vi "manage_objectives.vi"(8 "error in (no error)":errorcluster) -> (0 "error out":errorcluster)   [LabVIEW 2010]
uses:
  components/Objective/GenericObjective/GenericObjective/GenericObjective.lvclass
panel:
  in  "renameButton":bool
  in  "deleteButton":bool
  in  "editButton":bool
  in  "doneButton":bool
  in  "createButton":bool
  in  "new configuration":string
  in  "existing configurations":i32(listbox)
  # "Manage objectives"
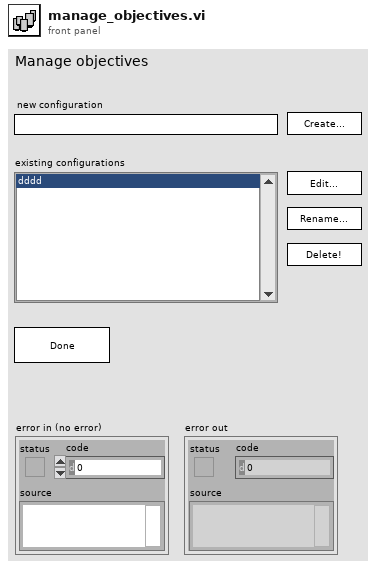
[diagram p1: front panel]
types:
  T1 = enum8{"Enabled", "Disabled", "Disabled and Grayed Out"}
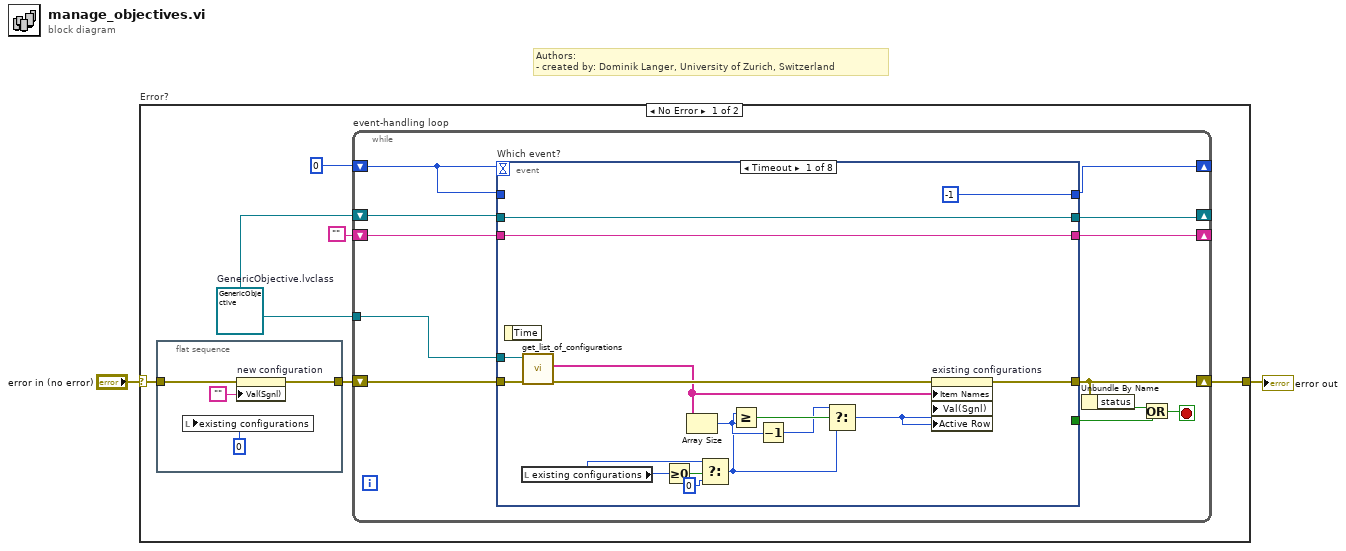
[diagram p0: block diagram]
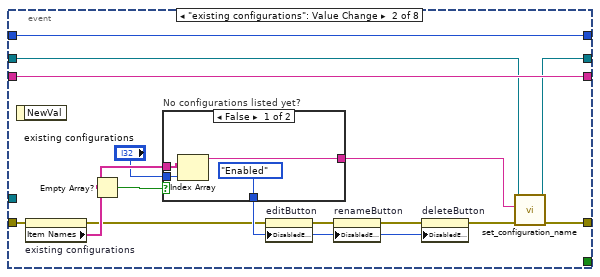
[diagram p2: hidden frame]
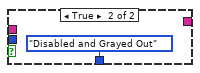
[diagram p3: hidden frame]
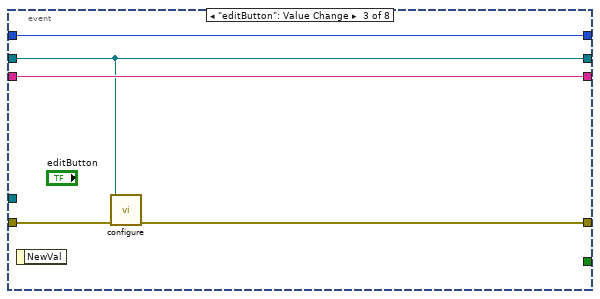
[diagram p4: hidden frame]
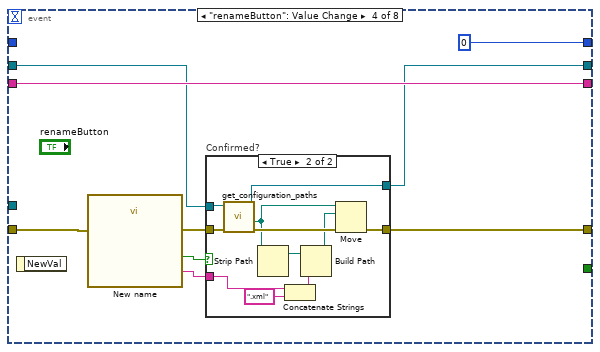
[diagram p5: hidden frame]
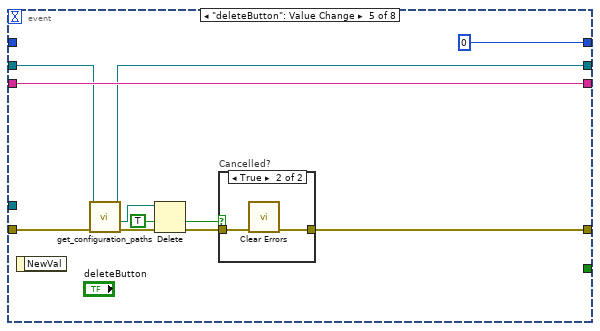
[diagram p7: hidden frame]
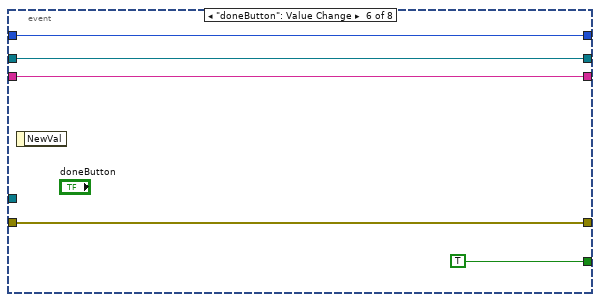
[diagram p9: hidden frame]
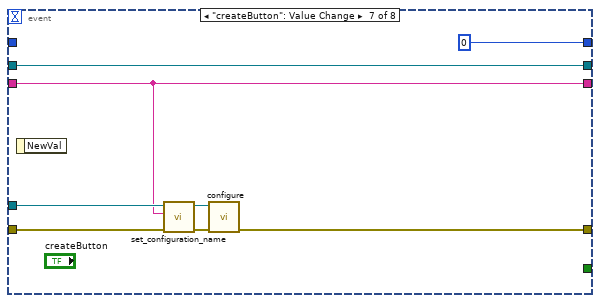
[diagram p10: hidden frame]
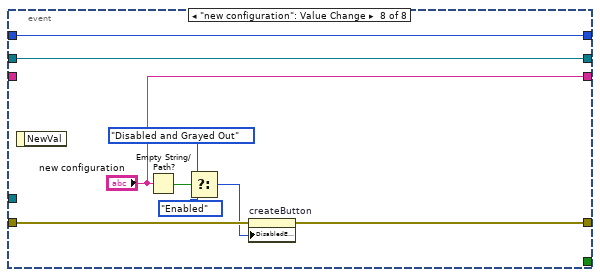
[diagram p11: hidden frame]
diagram:
  # "Authors: \n- created by: Dominik Langer, University of Zurich, Switzerland"
  n1 = case "Error?" shown="No Error" "error in (no error)" {
    selector: "error in (no error)" -> [w6 w124]
    tunnel: [w8 w124] -> w1
    frame No Error {
      w3 = refnum<class "GenericObjective.lvclass"> refnum  # GenericObjective.lvclass
      n2 = flat-sequence {
        tunnel: w6 -> [w12]
        tunnel: [w11] -> w5
        frame #0 {
          n3 = local write "existing configurations"(0) -> ()
          n4 = property on="new configuration" class="Str"(error in=w12, "Val(Sgnl)"="") -> (error out=w11:errorcluster)  [unwired: 1 in, 1 out]
        }
      }
      n5 = while "event-handling loop" {
        shift-right: [w23] -> w8
        shift-left: w5 -> [w24]
        shift-right: [w18] -> _
        shift-left: 0 -> [w19]
        tunnel: w3 -> [w17]
        shift-right: [w15] -> _
        shift-left: w3 -> [w16]
        shift-right: [w14] -> _
        shift-left: "" -> [w13]
        stop <- w21 stop-if-true
        n6 = event "Which event?" shown="[0] Timeout" {
          selector: _ -> [_ _ _ _ _ _ _ _]
          dyn-events: _ -> [_ _ _ _ _ _ _ _]
          timeout: w19 -> [_ _ _ _ _ _ _ _]
          tunnel: w24 -> [w38 w53 w62 w72 w96 w106 w113 w121]
          tunnel: [w36 w44 w63 w68 w89 w106 w114 w120] -> w23
          tunnel: [_ _ _ _ _ TRUE _ _] -> w20
          tunnel: [-1 w55 w65 0 0 w104 0 w123] -> w18
          tunnel: w19 -> [_ w55 w65 _ _ w104 _ w123]
          tunnel: w17 -> [w39 _ _ _ _ _ w109 _]
          tunnel: w16 -> [w35 w43 w61 w70 w95 w103 w108 w122]
          tunnel: [w35 w42 w61 w69 w94 w103 w108 w122] -> w15
          tunnel: [w34 w54 w64 w73 w97 w102 w107 "new configuration"] -> w14
          tunnel: w13 -> [w34 w54 w64 w73 w97 w102 w107 _]
          event Timeout {
            n7 = event-data() -> ()  [unwired: 1 in, 1 out]
            n8 = local read "existing configurations"() -> (w27:i32)
            n9 = call-dynamic "get_list_of_configurations.vi"("error in (no error)"=w38, "GenericComponent in"=w39) -> ("error out"=w37:errorcluster, "configurations"=w33:string[])  [unwired: 7 in, 1 out]
            n10 = Greater Or Equal To 0?(x=w27) -> (x >= 0?=w28:bool)
            n11 = Array Size(array=w33) -> (size(s)=w31:i32)
            n12 = Select(t=w27, s=w28, f=0) -> (s? t:f=w26:i32)
            n13 = Greater Or Equal?(x=w26, y=w31) -> (x >= y?=w32:bool)
            n14 = Decrement(x=w31) -> (x-1=w30:i32)
            n15 = Select(t=w30, s=w32, f=w26) -> (s? t:f=w29:i32)
            n16 = property on="existing configurations" class="LstBox (strict)"(error in=w37, "Item Names"=w33, "Val(Sgnl)"=w29, "Active Row"=w29) -> (error out=w36:errorcluster)  [unwired: 1 in, 1 out]
          }
          event "existing configurations": Value Change {
            n17 = event-data() -> ()  [unwired: 1 in, 1 out]
            n18 = property on="existing configurations" class="LstBox (strict)"(error in=w53) -> (error out=w46:errorcluster, "Item Names"=w52:string[])  [unwired: 1 in, 1 out]
            n19 = Empty Array?(array=w52) -> (empty?=w51:bool)
            n20 = case "No configurations listed yet?" shown="False" w51 {
              tunnel: [w59 _] -> w41
              tunnel: w52 -> [w58 _]
              tunnel: "existing configurations" -> [w57 _]
              tunnel: [T1."Enabled" ("Disabled") T1."Disabled and Grayed Out" ("Disabled")] -> w47
              frame False {
                n21 = Index Array(array=w58, index=w57) -> (element=w59:string)
              }
              frame True {
              }
            }
            n22 = property on="editButton" class="Bool"(error in=w46, "DisabledEnum"=w47) -> (error out=w49:errorcluster)  [unwired: 1 in, 1 out]
            n23 = property on="renameButton" class="Bool"(error in=w49, "DisabledEnum"=w47) -> (error out=w48:errorcluster)  [unwired: 1 in, 1 out]
            n24 = property on="deleteButton" class="Bool"(error in=w48, "DisabledEnum"=w47) -> (error out=w45:errorcluster)  [unwired: 1 in, 1 out]
            n25 = call-dynamic "set_configuration_name.vi"("error in (no error)"=w45, "configuration"=w41, "GenericPlugin.lvclass in"=w43) -> ("error out"=w44:errorcluster, "GenericPlugin.lvclass out"=w42:refnum<class "GenericObjective.lvclass">)  [unwired: 7 in]
          }
          event "editButton": Value Change {
            n26 = event-data() -> ()  [unwired: 1 in, 1 out]
            n27 = call-dynamic "configure.vi"("error in (no error)"=w62, "GenericObjective in"=w61) -> ("error out"=w63:errorcluster)  [unwired: 8 in, 1 out]
          }
          event "renameButton": Value Change {
            n28 = event-data() -> ()  [unwired: 1 in, 1 out]
            n29 = call "New name"("error in (no error)"=w72) -> ("New name"=w66:string, "OK"=w67:bool, "error out"=w71:errorcluster)  [unwired: 16 in]
            n30 = case "Confirmed?" shown="True" w67 {
              tunnel: w71 -> [w75 w87]
              tunnel: w70 -> [w76 w86]
              tunnel: [w76 w85] -> w69
              tunnel: [w75 w83] -> w68
              tunnel: w66 -> [_ w81]
              frame False {
              }
              frame True {
                n31 = call-dynamic "get_configuration_paths.vi"("error in (no error)"=w87, "GenericComponent in"=w86) -> ("error out"=w84:errorcluster, "configuration file path"=w79:path, "GenericComponent out"=w85:refnum<class "GenericObjective.lvclass">)  [unwired: 2 in, 5 out]
                n32 = Strip Path(path=w79) -> (stripped path=w82:path)  [unwired: 1 out]
                n33 = Concatenate Strings(w81, ".xml" ("string")) -> (w80:string)
                n34 = Build Path(base path=w82, name or relative path=w80) -> (appended path=w77:path)
                n35 = Move(source path=w79, error in=w84, 10:w77) -> (error out=w83:errorcluster)  [unwired: 2 in, 2 out]
              }
            }
          }
          event "deleteButton": Value Change {
            n36 = event-data() -> ()  [unwired: 1 in, 1 out]
            n37 = call-dynamic "get_configuration_paths.vi"("error in (no error)"=w96, "GenericComponent in"=w95) -> ("error out"=w93:errorcluster, "configuration file path"=w92:path, "GenericComponent out"=w94:refnum<class "GenericObjective.lvclass">)  [unwired: 2 in, 5 out]
            n38 = Delete(path (use dialog)=w92, confirm (F)=TRUE, error in=w93) -> (cancelled=w88:bool, error out=w90:errorcluster)  [unwired: 2 in, 1 out]
            n39 = case "Cancelled?" shown="True" w88 {
              tunnel: w90 -> [w99 w101]
              tunnel: [w99 w100] -> w89
              frame False {
              }
              frame True {
                n40 = call <vilib>:"Clear Errors.vi"("error in (no error)"=w101) -> ("error out"=w100:errorcluster)  [unwired: 6 in]
              }
            }
          }
          event "doneButton": Value Change {
            n41 = event-data() -> ()  [unwired: 1 in, 1 out]
          }
          event "createButton": Value Change {
            n42 = event-data() -> ()  [unwired: 1 in, 1 out]
            n43 = call-dynamic "set_configuration_name.vi"("error in (no error)"=w113, "configuration"=w107, "GenericPlugin.lvclass in"=w109) -> ("error out"=w112:errorcluster, "GenericPlugin.lvclass out"=w111:refnum<class "GenericObjective.lvclass">)  [unwired: 7 in]
            n44 = call-dynamic "configure.vi"("error in (no error)"=w112, "GenericObjective in"=w111) -> ("error out"=w114:errorcluster)  [unwired: 8 in, 1 out]
          }
          event "new configuration": Value Change {
            n45 = event-data() -> ()  [unwired: 1 in, 1 out]
            n46 = Empty String/Path?(string/path="new configuration") -> (empty?=w119:bool)
            n47 = Select(t=T1."Disabled and Grayed Out", s=w119, f=T1."Enabled" ("Disabled")) -> (s? t:f=w117:T1)
            n48 = property on="createButton" class="Bool"(error in=w121, "DisabledEnum"=w117) -> (error out=w120:errorcluster)  [unwired: 1 in, 1 out]
          }
        }
        n49 = Unbundle By Name(w23) -> ("status"=w22:bool)
        n50 = Or(x=w22, y=w20) -> (x .or. y?=w21:bool)
      }
    }
    frame Error {
    }
  }
  "error out" <- w1
